vi "Create Test Configuration.vi"() -> (0 "error out":errorcluster, 1 "Names":string[](array[string]), 2 "Line Array":T1(array[cluster]), 3 "Module":refnum<class "DAQmx Watchdog configuration.lvclass">, 4 "Channels":refnum<class "TBM channel.lvclass">[](array[class]), 5 "instance identifier":string)   [LabVIEW 2014, in "DAQmx Watchdog tests.lvlib"]
uses:
  DAQmx Watchdog tests.lvlib
  <vilib>/NI/Tag Bus Module Framework/channel/TBM channel.lvclass
  module/configuration/DAQmx Watchdog configuration.lvclass
  <vilib>/NI/Tag Bus/tag/tag descriptor.lvclass/tag descriptor.ctl
  <vilib>/NI/DCAF/Tag Editor Core/control module/configuration/control module configuration.lvclass/control module configuration.ctl
  <vilib>/NI/Tag Bus/tag/read tag name.vi
  <vilib>/NI/DCAF/Tag Editor Core/control module/configuration/Write configured channels.vi
  <vilib>/NI/Configuration Framework/serializable configuration/NISE_CEF_serializable configuration.lvclass
  <vilib>/NI/DCAF/Tag Editor Core/control module/configuration/control module configuration.lvclass
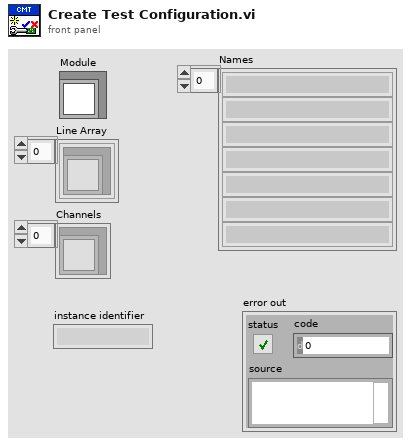
[diagram p1: front panel]
types:
  T1 = cluster{"channel":refnum<class "TBM channel.lvclass">}[]
  T2 = cluster{"physical channel(s)":tag, "expiration state":i32}[]
  T3 = cluster{"physical channel":tag, "expiration state":dbl, "output type":i32}[]
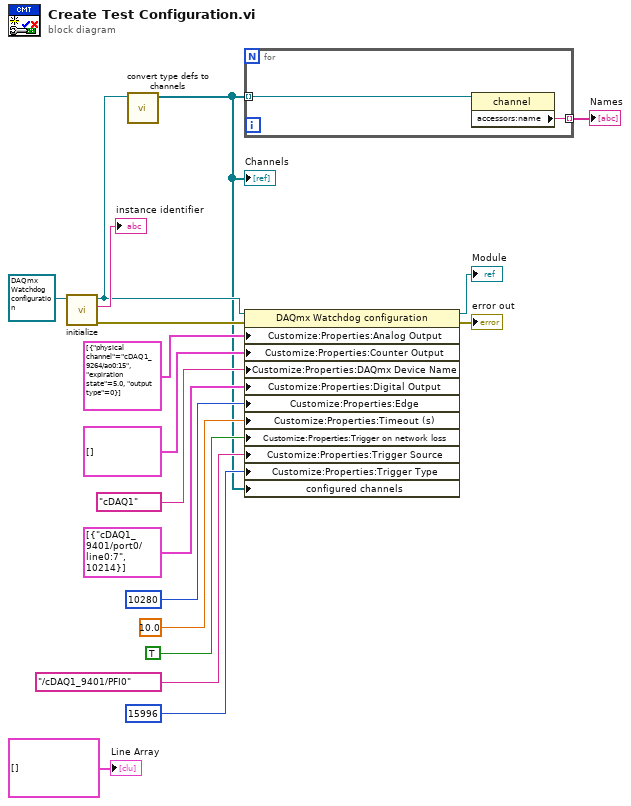
[diagram p0: block diagram]
diagram:
  n1 = call <vilib>:"initialize.vi"("configuration in"=refnum<class "DAQmx Watchdog configuration.lvclass"> refnum ("user control module configuration")) -> ("error out"=w17:errorcluster, "identifier"=→"instance identifier":string, "configuration out"=w3:refnum<class "DAQmx Watchdog configuration.lvclass">)  [unwired: 8 in]
  n2 = call <vilib>:"convert type defs to channels.vi"("fixed channel configuration"=w3) -> ("Array out"=w2:refnum<class "TBM channel.lvclass">[])  [unwired: 9 in, 1 out]
  "Channels" <- w2
  n3 = for {
    tunnel: w2 -> [w20] mode=indexing
    tunnel: [w19] -> w1 mode=indexing
    n4 = property class="channel"(reference=w20) -> ("accessors:name"=w19:string)  [unwired: 1 in, 2 out]
  }
  "Names" <- w1
  n5 = property class="DAQmx Watchdog configuration"(reference=w3, error in=w17, "Customize:Properties:Analog Output"=T3 [{"physical channel"="cDAQ1_9264/ao0:15", "expiration state"=5.0, "output type"=0}] ("Analog Output"), "Customize:Properties:Counter Output"=T2 [] ("Counter Output"), "Customize:Properties:DAQmx Device Name"=tag "cDAQ1" ("DAQmx Device Name"), "Customize:Properties:Digital Output"=T2 [{"physical channel(s)"="cDAQ1_9401/port0/line0:7", "expiration state"=10214}] ("Digital Output"), "Customize:Properties:Edge"=10280 ("Edge"), "Customize:Properties:Timeout (s)"=10.0 ("Timeout (s)"), "Customize:Properties:Trigger on network loss"=TRUE ("Trigger on network loss"), "Customize:Properties:Trigger Source"=tag "/cDAQ1_9401/PFI0" ("Trigger Source"), "Customize:Properties:Trigger Type"=15996 ("Trigger Type"), "configured channels"=w2) -> (reference out=→"Module":refnum<class "DAQmx Watchdog configuration.lvclass">, error out=→"error out":errorcluster)
  "Line Array" <- T1 [] ("Line Array")
